vi "traffic control puls.vi"(7 "state":u16(ring) items=["Init", "Get"], 11 "blinke periode (s)":u32=2) -> (3 "puls":bool)   [LabVIEW 2017]
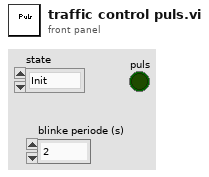
[diagram p1: front panel]
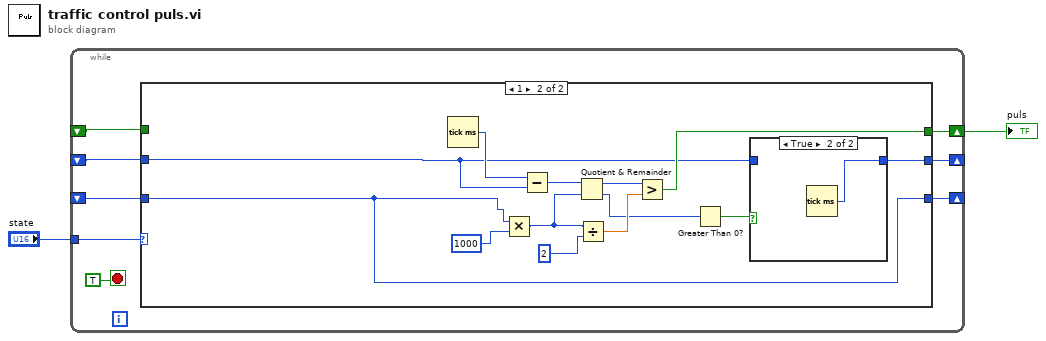
[diagram p0: block diagram]
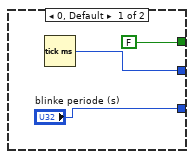
[diagram p2: hidden frame]
diagram:
  n1 = while {
    shift-right: [w10] -> w1
    shift-left: _ -> [w8]
    shift-right: [w9] -> _
    shift-left: _ -> [w7]
    tunnel: "state" -> [w6]
    shift-right: [w4] -> _
    shift-left: _ -> [w3]
    stop <- TRUE stop-if-true
    n2 = case shown="1" w6 {
      tunnel: [FALSE ("Boolean") w19] -> w10
      tunnel: [w12 w16] -> w9
      tunnel: w8 -> [_ _]
      tunnel: w7 -> [_ w15]
      tunnel: ["blinke periode (s)" w14] -> w4
      tunnel: w3 -> [_ w14]
      frame 0, Default {
        n3 = Tick Count (ms)() -> (millisecond timer value=w12:u32)
      }
      frame 1 {
        n4 = Tick Count (ms)() -> (millisecond timer value=w23:u32)
        n5 = Multiply(x=w14, y=u32 1000) -> (x*y=w22:u32)
        n6 = Subtract(x=w23, y=w15) -> (x-y=w26:u32)
        n7 = Quotient & Remainder(x=w26, y=w22) -> (x-y*floor(x/y)=w25:u32, floor(x/y)=w18:u32)
        n8 = Divide(x=w22, y=u32 2) -> (x/y=w24:dbl)
        n9 = Greater?(x=w25, y=w24) -> (0:w19:bool)
        n10 = Greater Than 0?(x=w18) -> (x > 0?=w17:bool)
        n11 = case shown="True" w17 {
          tunnel: [w27 w28] -> w16
          tunnel: w15 -> [w27 _]
          frame False {
          }
          frame True {
            n12 = Tick Count (ms)() -> (millisecond timer value=w28:u32)
          }
        }
      }
    }
  }
  "puls" <- w1
